vi "Setup Data.vi"(11 "?":T2={"Input Data 1D"=[], "Channel Settings"={"Supply Voltage [Vdc]"=0.0, "Max Supply Current [Idc]"=0.0, "Settling Delay"=0.0, "Temp Criteria"=0.0, "Voltage Steps [Vrms]"=[0.0, 0.25, 0.5, 1.0, 1.95, 3.0, 3.9, 5.5], "User Notes"="", "Config Wave File Path"=path "C:/ASD Power Point Beta 32J/Waveforms/150HzSine5Second.wav", "Config Voltage [Vrms]"=0.0, "Channel Configuration List"={"Channel Configuration Cluster"={"Input"=enum."---", "Enable"=FALSE, "User Notes"="", "Voltage Range"=0.0, "Current Range"=2.5}, "Channel Configuration Cluster 2"={"Input"=enum."---", "Enable"=FALSE, "User Notes"="", "Voltage Range"=0.0, "Current Range"=2.5}, "Channel Configuration Cluster 3"={"Input"=enum."---", "Enable"=FALSE, "User Notes"="", "Voltage Range"=0.0, "Current Range"=2.5}, "Channel Configuration Cluster 4"={"Input"=enum."---", "Enable"=FALSE, "User Notes"="", "Voltage Range"=0.0, "Current Range"=2.5}, "Channel Configuration Cluster 5"={"Input"=enum."---", "Enable"=FALSE, "User Notes"="", "Voltage Range"=0.0, "Current Range"=2.5}, "Channel Configuration Cluster 6"={"Input"=enum."---", "Enable"=FALSE, "User Notes"="", "Voltage Range"=0.0, "Current Range"=2.5}, "Channel Configuration Cluster 7"={"Input"=enum."---", "Enable"=FALSE, "User Notes"="", "Voltage Range"=0.0, "Current Range"=2.5}, "Channel Configuration Cluster 8"={"Input"=enum."---", "Enable"=FALSE, "User Notes"="", "Voltage Range"=0.0, "Current Range"=2.5}, "Channel Configuration Cluster 9"={"Input"=enum."---", "Enable"=FALSE, "User Notes"="", "Voltage Range"=0.0, "Current Range"=2.5}, "Channel Configuration Cluster 10"={"Input"=enum."---", "Enable"=FALSE, "User Notes"="", "Voltage Range"=0.0, "Current Range"=2.5}, "Channel Configuration Cluster 11"={"Input"=enum."---", "Enable"=FALSE, "User Notes"="", "Voltage Range"=0.0, "Current Range"=2.5}, "Channel Configuration Cluster 12"={"Input"=enum."---", "Enable"=FALSE, "User Notes"="", "Voltage Range"=0.0, "Current Range"=2.5}, "Channel Configuration Cluster 13"={"Input"=enum."---", "Enable"=FALSE, "User Notes"="", "Voltage Range"=0.0, "Current Range"=2.5}, "Channel Configuration Cluster 14"={"Input"=enum."---", "Enable"=FALSE, "User Notes"="", "Voltage Range"=0.0, "Current Range"=2.5}, "Channel Configuration Cluster 15"={"Input"=enum."---", "Enable"=FALSE, "User Notes"="", "Voltage Range"=0.0, "Current Range"=2.5}, "Channel Configuration Cluster 16"={"Input"=enum."---", "Enable"=FALSE, "User Notes"="", "Voltage Range"=0.0, "Current Range"=2.5}, "Channel Configuration Cluster 17"={"Input"=enum."---", "Enable"=FALSE, "User Notes"="", "Voltage Range"=0.0, "Current Range"=2.5}}, "User Gains"={"Gain 1"=0.0, "Gain 2"=0.0, "Gain 3"=0.0, "Gain 4"=0.0, "Gain 5"=0.0, "Gain 6"=0.0}, "Gains"={"Gain 1"=0.0, "Gain 2"=0.0, "Gain 3"=0.0, "Gain 4"=0.0, "Gain 5"=0.0, "Gain 6"=0.0}, "Gain Array"={"Gain 1"=0.0, "Gain 2"=0.0, "Gain 3"=0.0, "Gain 4"=0.0, "Gain 5"=0.0, "Gain 6"=0.0, "Gain 7"=0.0, "Gain 8"=0.0, "Gain 9"=0.0, "Gain 10"=0.0, "Gain 11"=0.0, "Gain 12"=0.0, "Gain 13"=0.0, "Gain 14"=0.0, "Gain 15"=0.0, "Gain 16"=0.0, "Gain 17"=0.0}, "Wave File Path 1"=path "", "Wave File Path 2"=path "", "Wave File Path 3"=path "", "Wave File Path 4"=path "", "Range"=FALSE, "CF"=FALSE}, "Select Data"={"Vrms Data"=FALSE, "Vpkpk Data"=FALSE, "Irms Data"=FALSE, "Power Data"=FALSE, "Ipkpk Data"=FALSE, "Temp Data"=FALSE}, "Detailed Report ?"=FALSE, "Path Settings:"={"Template Path "=path "E:/L&T Projects/Bose ASD/Excel Template/ASD Template.xltx", "Report Path"=path "E:/L&T Projects/Bose ASD/excel Reports", "JPEG1 Path "=path "C:/Users/Public/Pictures/Sample Pictures/Hydrangeas.jpg", "JPEG2 Path"=path "C:/Users/Public/Pictures/Sample Pictures/Lighthouse.jpg"}, "Vrms_Sheet"=[], "Irms_Sheet"=[], "Power_Sheet"=[], "Vpk_Sheet"=[], "Ipk_Sheet"=[], "Vrms_Avg"=[], "Irms_Avg"=[], "Power_Avg"=[], "Vpk_Avg"=[], "Ipk_Avg"=[], "Report_Ref"=refnum, "User Name"="", "Temp_Sheet"=[]} {"Channel Settings"."Gain Array"."Gain 17" format="%.2f"; "Channel Settings"."Gain Array"."Gain 16" format="%.2f"; "Channel Settings"."Gain Array"."Gain 15" format="%.2f"; "Channel Settings"."Gain Array"."Gain 14" format="%.2f"; "Channel Settings"."Gain Array"."Gain 13" format="%.2f"; "Channel Settings"."Gain Array"."Gain 12" format="%.2f"; "Channel Settings"."Gain Array"."Gain 11" format="%.2f"; "Channel Settings"."Gain Array"."Gain 10" format="%.2f"; "Channel Settings"."Gain Array"."Gain 9" format="%.2f"; "Channel Settings"."Gain Array"."Gain 8" format="%.2f"; "Channel Settings"."Gain Array"."Gain 7" format="%.2f"; "Channel Settings"."Gain Array"."Gain 6" format="%.2f"; "Channel Settings"."Gain Array"."Gain 5" format="%.2f"; "Channel Settings"."Gain Array"."Gain 4" format="%.2f"; "Channel Settings"."Gain Array"."Gain 3" format="%.2f"; "Channel Settings"."Gain Array"."Gain 2" format="%.2f"; "Channel Settings"."Gain Array"."Gain 1" format="%.2f"; "Channel Settings"."Gains"."Gain 6" format="%.2f"; "Channel Settings"."Gains"."Gain 5" format="%.2f"; "Channel Settings"."Gains"."Gain 4" format="%.2f"; "Channel Settings"."Gains"."Gain 3" format="%.2f"; "Channel Settings"."Gains"."Gain 2" format="%.2f"; "Channel Settings"."Gains"."Gain 1" format="%.2f"; "Channel Settings"."User Gains"."Gain 6" format="%.2f"; "Channel Settings"."User Gains"."Gain 5" format="%.2f"; "Channel Settings"."User Gains"."Gain 4" format="%.2f"; "Channel Settings"."User Gains"."Gain 3" format="%.2f"; "Channel Settings"."User Gains"."Gain 2" format="%.2f"; "Channel Settings"."User Gains"."Gain 1" format="%.2f"; "Channel Settings"."Channel Configuration List"."Channel Configuration Cluster 17"."Current Range" items=["1 <500m>"=0.5, "2 <1>"=1.0, "5 <2.5>"=2.5, "10 <5>"=5.0, "20 <10>"=10.0, "50 <25>"=25.0]; "Channel Settings"."Channel Configuration List"."Channel Configuration Cluster 17"."Voltage Range" items=["1.5 <0.75>"=0.75, "3 <1.5>"=1.5, "6 <3>"=3.0, "10 <5>"=5.0, "15 <7.5>"=7.5, "30 <15>"=15.0, "60 <30>"=30.0, "100 <50>"=50.0, "150 <75>"=75.0, "300 <150>"=150.0, "600 <300>"=300.0, "1000 <500>"=500.0]; "Channel Settings"."Channel Configuration List"."Channel Configuration Cluster 16"."Current Range" items=["1 <500m>"=0.5, "2 <1>"=1.0, "5 <2.5>"=2.5, "10 <5>"=5.0, "20 <10>"=10.0, "50 <25>"=25.0]; "Channel Settings"."Channel Configuration List"."Channel Configuration Cluster 16"."Voltage Range" items=["1.5 <0.75>"=0.75, "3 <1.5>"=1.5, "6 <3>"=3.0, "10 <5>"=5.0, "15 <7.5>"=7.5, "30 <15>"=15.0, "60 <30>"=30.0, "100 <50>"=50.0, "150 <75>"=75.0, "300 <150>"=150.0, "600 <300>"=300.0, "1000 <500>"=500.0]; "Channel Settings"."Channel Configuration List"."Channel Configuration Cluster 15"."Current Range" items=["1 <500m>"=0.5, "2 <1>"=1.0, "5 <2.5>"=2.5, "10 <5>"=5.0, "20 <10>"=10.0, "50 <25>"=25.0]; "Channel Settings"."Channel Configuration List"."Channel Configuration Cluster 15"."Voltage Range" items=["1.5 <0.75>"=0.75, "3 <1.5>"=1.5, "6 <3>"=3.0, "10 <5>"=5.0, "15 <7.5>"=7.5, "30 <15>"=15.0, "60 <30>"=30.0, "100 <50>"=50.0, "150 <75>"=75.0, "300 <150>"=150.0, "600 <300>"=300.0, "1000 <500>"=500.0]; "Channel Settings"."Channel Configuration List"."Channel Configuration Cluster 14"."Current Range" items=["1 <500m>"=0.5, "2 <1>"=1.0, "5 <2.5>"=2.5, "10 <5>"=5.0, "20 <10>"=10.0, "50 <25>"=25.0]; "Channel Settings"."Channel Configuration List"."Channel Configuration Cluster 14"."Voltage Range" items=["1.5 <0.75>"=0.75, "3 <1.5>"=1.5, "6 <3>"=3.0, "10 <5>"=5.0, "15 <7.5>"=7.5, "30 <15>"=15.0, "60 <30>"=30.0, "100 <50>"=50.0, "150 <75>"=75.0, "300 <150>"=150.0, "600 <300>"=300.0, "1000 <500>"=500.0]; "Channel Settings"."Channel Configuration List"."Channel Configuration Cluster 13"."Current Range" items=["1 <500m>"=0.5, "2 <1>"=1.0, "5 <2.5>"=2.5, "10 <5>"=5.0, "20 <10>"=10.0, "50 <25>"=25.0]; "Channel Settings"."Channel Configuration List"."Channel Configuration Cluster 13"."Voltage Range" items=["1.5 <0.75>"=0.75, "3 <1.5>"=1.5, "6 <3>"=3.0, "10 <5>"=5.0, "15 <7.5>"=7.5, "30 <15>"=15.0, "60 <30>"=30.0, "100 <50>"=50.0, "150 <75>"=75.0, "300 <150>"=150.0, "600 <300>"=300.0, "1000 <500>"=500.0]; "Channel Settings"."Channel Configuration List"."Channel Configuration Cluster 12"."Current Range" items=["1 <500m>"=0.5, "2 <1>"=1.0, "5 <2.5>"=2.5, "10 <5>"=5.0, "20 <10>"=10.0, "50 <25>"=25.0]; "Channel Settings"."Channel Configuration List"."Channel Configuration Cluster 12"."Voltage Range" items=["1.5 <0.75>"=0.75, "3 <1.5>"=1.5, "6 <3>"=3.0, "10 <5>"=5.0, "15 <7.5>"=7.5, "30 <15>"=15.0, "60 <30>"=30.0, "100 <50>"=50.0, "150 <75>"=75.0, "300 <150>"=150.0, "600 <300>"=300.0, "1000 <500>"=500.0]; "Channel Settings"."Channel Configuration List"."Channel Configuration Cluster 11"."Current Range" items=["1 <500m>"=0.5, "2 <1>"=1.0, "5 <2.5>"=2.5, "10 <5>"=5.0, "20 <10>"=10.0, "50 <25>"=25.0]; "Channel Settings"."Channel Configuration List"."Channel Configuration Cluster 11"."Voltage Range" items=["1.5 <0.75>"=0.75, "3 <1.5>"=1.5, "6 <3>"=3.0, "10 <5>"=5.0, "15 <7.5>"=7.5, "30 <15>"=15.0, "60 <30>"=30.0, "100 <50>"=50.0, "150 <75>"=75.0, "300 <150>"=150.0, "600 <300>"=300.0, "1000 <500>"=500.0]; "Channel Settings"."Channel Configuration List"."Channel Configuration Cluster 10"."Current Range" items=["1 <500m>"=0.5, "2 <1>"=1.0, "5 <2.5>"=2.5, "10 <5>"=5.0, "20 <10>"=10.0, "50 <25>"=25.0]; "Channel Settings"."Channel Configuration List"."Channel Configuration Cluster 10"."Voltage Range" items=["1.5 <0.75>"=0.75, "3 <1.5>"=1.5, "6 <3>"=3.0, "10 <5>"=5.0, "15 <7.5>"=7.5, "30 <15>"=15.0, "60 <30>"=30.0, "100 <50>"=50.0, "150 <75>"=75.0, "300 <150>"=150.0, "600 <300>"=300.0, "1000 <500>"=500.0]; "Channel Settings"."Channel Configuration List"."Channel Configuration Cluster 9"."Voltage Range" items=["1.5 <0.75>"=0.75, "3 <1.5>"=1.5, "6 <3>"=3.0, "10 <5>"=5.0, "15 <7.5>"=7.5, "30 <15>"=15.0, "60 <30>"=30.0, "100 <50>"=50.0, "150 <75>"=75.0, "300 <150>"=150.0, "600 <300>"=300.0, "1000 <500>"=500.0]; "Channel Settings"."Channel Configuration List"."Channel Configuration Cluster 9"."Current Range" items=["10m <5m>"=0.005, "20m <10m>"=0.01, "50m <25m>"=0.025, "100m <50m>"=0.05, "200m <100m>"=0.1, "500m <250m>"=0.25, "1 <500m>"=0.5, "2 <1>"=1.0, "5 <2.5>"=2.5]; "Channel Settings"."Channel Configuration List"."Channel Configuration Cluster 8"."Voltage Range" items=["1.5 <0.75>"=0.75, "3 <1.5>"=1.5, "6 <3>"=3.0, "10 <5>"=5.0, "15 <7.5>"=7.5, "30 <15>"=15.0, "60 <30>"=30.0, "100 <50>"=50.0, "150 <75>"=75.0, "300 <150>"=150.0, "600 <300>"=300.0, "1000 <500>"=500.0]; "Channel Settings"."Channel Configuration List"."Channel Configuration Cluster 8"."Current Range" items=["10m <5m>"=0.005, "20m <10m>"=0.01, "50m <25m>"=0.025, "100m <50m>"=0.05, "200m <100m>"=0.1, "500m <250m>"=0.25, "1 <500m>"=0.5, "2 <1>"=1.0, "5 <2.5>"=2.5]; "Channel Settings"."Channel Configuration List"."Channel Configuration Cluster 7"."Voltage Range" items=["1.5 <0.75>"=0.75, "3 <1.5>"=1.5, "6 <3>"=3.0, "10 <5>"=5.0, "15 <7.5>"=7.5, "30 <15>"=15.0, "60 <30>"=30.0, "100 <50>"=50.0, "150 <75>"=75.0, "300 <150>"=150.0, "600 <300>"=300.0, "1000 <500>"=500.0]; "Channel Settings"."Channel Configuration List"."Channel Configuration Cluster 7"."Current Range" items=["10m <5m>"=0.005, "20m <10m>"=0.01, "50m <25m>"=0.025, "100m <50m>"=0.05, "200m <100m>"=0.1, "500m <250m>"=0.25, "1 <500m>"=0.5, "2 <1>"=1.0, "5 <2.5>"=2.5]; "Channel Settings"."Channel Configuration List"."Channel Configuration Cluster 6"."Voltage Range" items=["1.5 <0.75>"=0.75, "3 <1.5>"=1.5, "6 <3>"=3.0, "10 <5>"=5.0, "15 <7.5>"=7.5, "30 <15>"=15.0, "60 <30>"=30.0, "100 <50>"=50.0, "150 <75>"=75.0, "300 <150>"=150.0, "600 <300>"=300.0, "1000 <500>"=500.0]; "Channel Settings"."Channel Configuration List"."Channel Configuration Cluster 6"."Current Range" items=["10m <5m>"=0.005, "20m <10m>"=0.01, "50m <25m>"=0.025, "100m <50m>"=0.05, "200m <100m>"=0.1, "500m <250m>"=0.25, "1 <500m>"=0.5, "2 <1>"=1.0, "5 <2.5>"=2.5]; "Channel Settings"."Channel Configuration List"."Channel Configuration Cluster 5"."Voltage Range" items=["1.5 <0.75>"=0.75, "3 <1.5>"=1.5, "6 <3>"=3.0, "10 <5>"=5.0, "15 <7.5>"=7.5, "30 <15>"=15.0, "60 <30>"=30.0, "100 <50>"=50.0, "150 <75>"=75.0, "300 <150>"=150.0, "600 <300>"=300.0, "1000 <500>"=500.0]; "Channel Settings"."Channel Configuration List"."Channel Configuration Cluster 5"."Current Range" items=["10m <5m>"=0.005, "20m <10m>"=0.01, "50m <25m>"=0.025, "100m <50m>"=0.05, "200m <100m>"=0.1, "500m <250m>"=0.25, "1 <500m>"=0.5, "2 <1>"=1.0, "5 <2.5>"=2.5]; "Channel Settings"."Channel Configuration List"."Channel Configuration Cluster 4"."Voltage Range" items=["1.5 <0.75>"=0.75, "3 <1.5>"=1.5, "6 <3>"=3.0, "10 <5>"=5.0, "15 <7.5>"=7.5, "30 <15>"=15.0, "60 <30>"=30.0, "100 <50>"=50.0, "150 <75>"=75.0, "300 <150>"=150.0, "600 <300>"=300.0, "1000 <500>"=500.0]; "Channel Settings"."Channel Configuration List"."Channel Configuration Cluster 4"."Current Range" items=["10m <5m>"=0.005, "20m <10m>"=0.01, "50m <25m>"=0.025, "100m <50m>"=0.05, "200m <100m>"=0.1, "500m <250m>"=0.25, "1 <500m>"=0.5, "2 <1>"=1.0, "5 <2.5>"=2.5]; "Channel Settings"."Channel Configuration List"."Channel Configuration Cluster 3"."Voltage Range" items=["1.5 <0.75>"=0.75, "3 <1.5>"=1.5, "6 <3>"=3.0, "10 <5>"=5.0, "15 <7.5>"=7.5, "30 <15>"=15.0, "60 <30>"=30.0, "100 <50>"=50.0, "150 <75>"=75.0, "300 <150>"=150.0, "600 <300>"=300.0, "1000 <500>"=500.0]; "Channel Settings"."Channel Configuration List"."Channel Configuration Cluster 3"."Current Range" items=["10m <5m>"=0.005, "20m <10m>"=0.01, "50m <25m>"=0.025, "100m <50m>"=0.05, "200m <100m>"=0.1, "500m <250m>"=0.25, "1 <500m>"=0.5, "2 <1>"=1.0, "5 <2.5>"=2.5]; "Channel Settings"."Channel Configuration List"."Channel Configuration Cluster 2"."Voltage Range" items=["1.5 <0.75>"=0.75, "3 <1.5>"=1.5, "6 <3>"=3.0, "10 <5>"=5.0, "15 <7.5>"=7.5, "30 <15>"=15.0, "60 <30>"=30.0, "100 <50>"=50.0, "150 <75>"=75.0, "300 <150>"=150.0, "600 <300>"=300.0, "1000 <500>"=500.0]; "Channel Settings"."Channel Configuration List"."Channel Configuration Cluster 2"."Current Range" items=["10m <5m>"=0.005, "20m <10m>"=0.01, "50m <25m>"=0.025, "100m <50m>"=0.05, "200m <100m>"=0.1, "500m <250m>"=0.25, "1 <500m>"=0.5, "2 <1>"=1.0, "5 <2.5>"=2.5]; "Channel Settings"."Channel Configuration List"."Channel Configuration Cluster"."Voltage Range" items=["1.5 <0.75>"=0.75, "3 <1.5>"=1.5, "6 <3>"=3.0, "10 <5>"=5.0, "15 <7.5>"=7.5, "30 <15>"=15.0, "60 <30>"=30.0, "100 <50>"=50.0, "150 <75>"=75.0, "300 <150>"=150.0, "600 <300>"=300.0, "1000 <500>"=500.0]; "Channel Settings"."Channel Configuration List"."Channel Configuration Cluster"."Current Range" items=["10m <5m>"=0.005, "20m <10m>"=0.01, "50m <25m>"=0.025, "100m <50m>"=0.05, "200m <100m>"=0.1, "500m <250m>"=0.25, "1 <500m>"=0.5, "2 <1>"=1.0, "5 <2.5>"=2.5]; "Channel Settings"."Settling Delay" min=0.0 format="%<%H:%M:%S>t"; "Input Data 1D"."WT1800 Averages"."Vrms" format="%.3f"; "Input Data 1D"."WT1800 Averages"."Irms" format="%.3f"; "Input Data 1D"."WT1800 Averages"."Power" format="%.3f"; "Input Data 1D"."WT1800 Averages"."Vpkpk" format="%.3f"; "Input Data 1D"."WT1800 Averages"."Ipkpk" format="%.3f"; "Input Data 1D"."WT1800 Measurements"."Vrms" format="%.3f"; "Input Data 1D"."WT1800 Measurements"."Irms" format="%.3f"; "Input Data 1D"."WT1800 Measurements"."Power" format="%.3f"; "Input Data 1D"."WT1800 Measurements"."Vpkpk" format="%.3f"; "Input Data 1D"."WT1800 Measurements"."Ipkpk" format="%.3f"; "Input Data 1D"."DSA Averages"."Vrms" format="%.3f"; "Input Data 1D"."DSA Averages"."Vdc" format="%.3f"; "Input Data 1D"."DSA Averages"."Vpk+" format="%.3f"; "Input Data 1D"."DSA Averages"."Vpk-" format="%.3f"; "Input Data 1D"."DSA Averages"."Vpkpk" format="%.3f"; "Input Data 1D"."DSA Measurements"."Vrms" format="%.3f"; "Input Data 1D"."DSA Measurements"."Vdc" format="%.3f"; "Input Data 1D"."DSA Measurements"."Vpk+" format="%.3f"; "Input Data 1D"."DSA Measurements"."Vpk-" format="%.3f"; "Input Data 1D"."DSA Measurements"."Vpkpk" format="%.3f"}) -> (3 "Set up data":string[][][](array[string]))   [LabVIEW 2021]
uses:
  Datalog Controls/Data.ctl
  <vilib>/Utility/NIReport.llb/NI_report.lvclass
  Controls/Datalog Cluster Array.ctl
  Controls/Datalog Bundle Control.ctl
  Controls/WT1800 Functions.ctl
  Controls/WT1800 Measurements.ctl
  Controls/WT1800 Readings.ctl
  Controls/DSA Functions.ctl
  Controls/DSA Measurements.ctl
  Controls/DSA Readings.ctl
  Controls/Settings Control.ctl
  Controls/Channel Configuration List.ctl
  Controls/Channel Configuration Cluster.ctl
  Controls/Channel Configuration Cluster High Current.ctl
  Controls/Gain Averages.ctl
  Controls/Gain Array.ctl
  Datalog Controls/Select_Data.ctl
panel:
  out "Input":T1(ring)
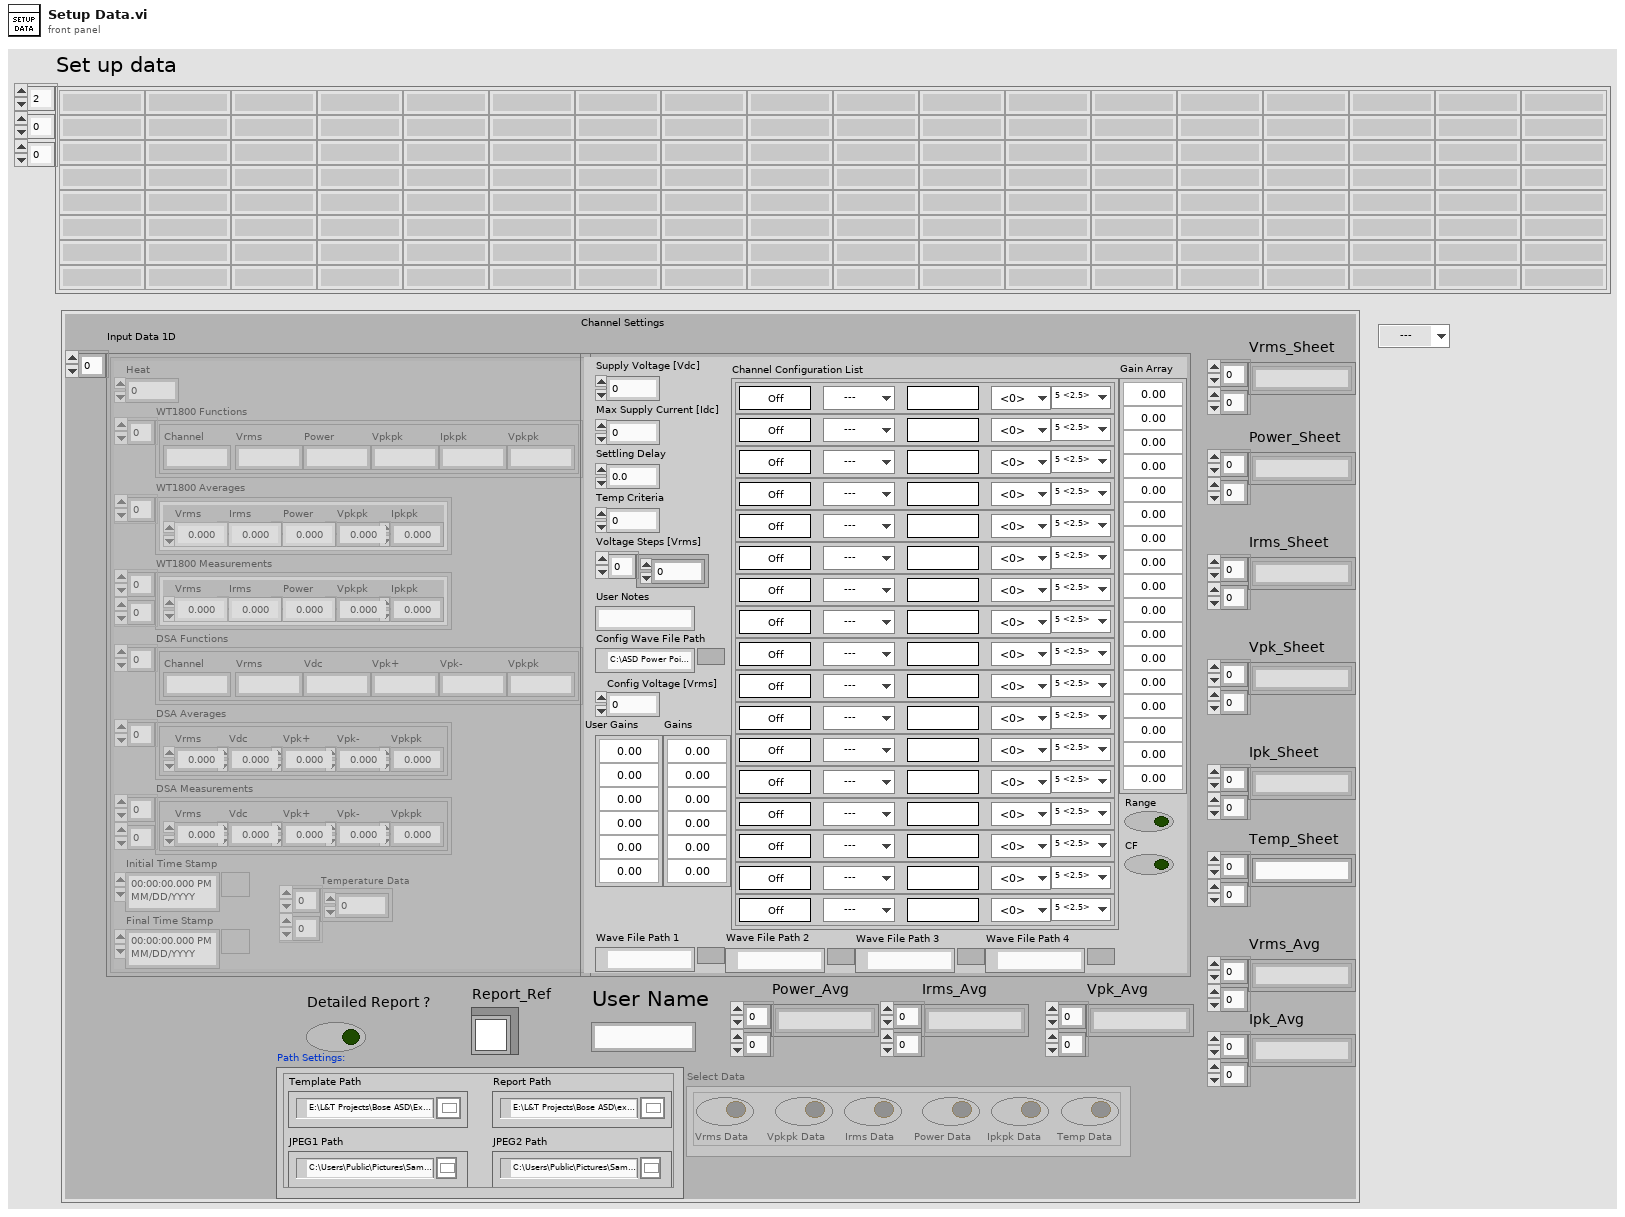
[diagram p1: front panel]
types:
  T1 = enum16{"---", "1", "1 AVG", "2", "2 AVG", "3", "3 AVG", "4", "4 AVG"}
  T2 = typedef "Data.ctl" = cluster{"Input Data 1D":T3, "Channel Settings":T11, "Select Data":T17, "Detailed Report ?":bool, "Path Settings:":cluster{"Template Path ":path, "Report Path":path, "JPEG1 Path ":path, "JPEG2 Path":path}, "Vrms_Sheet":string[][], "Irms_Sheet":string[][], "Power_Sheet":string[][], "Vpk_Sheet":string[][], "Ipk_Sheet":string[][], "Vrms_Avg":string[][], "Irms_Avg":string[][], "Power_Avg":string[][], "Vpk_Avg":string[][], "Ipk_Avg":string[][], "Report_Ref":refnum<class "NI_report.lvclass">, "User Name":string, "Temp_Sheet":string[][]}
  T3 = typedef "Datalog Cluster Array.ctl" = T4[]
  T4 = typedef "Datalog Bundle Control.ctl" = cluster{"Heat":dbl, "WT1800 Functions":T5, "WT1800 Averages":T6, "WT1800 Measurements":T7[][], "DSA Functions":T8, "DSA Averages":T9, "DSA Measurements":T10[][], "Initial Time Stamp":timestamp, "Final Time Stamp":timestamp, "Temperature Data":sgl[][]}
  T5 = typedef "WT1800 Functions.ctl" = cluster{"Channel":string, "Vrms":string, "Power":string, "Vpkpk":string, "Ipkpk":string, "Vpkpk":string}[]
  T6 = typedef "WT1800 Measurements.ctl" = T7[]
  T7 = typedef "WT1800 Readings.ctl" = cluster{"Vrms":sgl, "Irms":sgl, "Power":sgl, "Vpkpk":sgl, "Ipkpk":sgl}
  T8 = typedef "DSA Functions.ctl" = cluster{"Channel":string, "Vrms":string, "Vdc":string, "Vpk+":string, "Vpk-":string, "Vpkpk":string}[]
  T9 = typedef "DSA Measurements.ctl" = T10[]
  T10 = typedef "DSA Readings.ctl" = cluster{"Vrms":sgl, "Vdc":sgl, "Vpk+":sgl, "Vpk-":sgl, "Vpkpk":sgl}
  T11 = typedef "Settings Control.ctl" = cluster{"Supply Voltage [Vdc]":sgl, "Max Supply Current [Idc]":sgl, "Settling Delay":dbl, "Temp Criteria":sgl, "Voltage Steps [Vrms]":sgl[], "User Notes":string, "Config Wave File Path":path, "Config Voltage [Vrms]":sgl, "Channel Configuration List":T12, "User Gains":T15, "Gains":T15, "Gain Array":T16, "Wave File Path 1":path, "Wave File Path 2":path, "Wave File Path 3":path, "Wave File Path 4":path, "Range":bool, "CF":bool}
  T12 = typedef "Channel Configuration List.ctl" = cluster{"Channel Configuration Cluster":T13, "Channel Configuration Cluster 2":T13, "Channel Configuration Cluster 3":T13, "Channel Configuration Cluster 4":T13, "Channel Configuration Cluster 5":T13, "Channel Configuration Cluster 6":T13, "Channel Configuration Cluster 7":T13, "Channel Configuration Cluster 8":T13, "Channel Configuration Cluster 9":T13, "Channel Configuration Cluster 10":T14, "Channel Configuration Cluster 11":T14, "Channel Configuration Cluster 12":T14, "Channel Configuration Cluster 13":T14, "Channel Configuration Cluster 14":T14, "Channel Configuration Cluster 15":T14, "Channel Configuration Cluster 16":T14, "Channel Configuration Cluster 17":T14}
  T13 = typedef "Channel Configuration Cluster.ctl" = cluster{"Input":enum16{"---", "1", "1 AVG", "2", "2 AVG", "3", "3 AVG", "4", "4 AVG"}, "Enable":bool, "User Notes":string, "Voltage Range":dbl, "Current Range":dbl}
  T14 = typedef "Channel Configuration Cluster High Current.ctl" = cluster{"Input":enum16{"---", "1", "1 AVG", "2", "2 AVG", "3", "3 AVG", "4", "4 AVG"}, "Enable":bool, "User Notes":string, "Voltage Range":dbl, "Current Range":dbl}
  T15 = typedef "Gain Averages.ctl" = cluster{"Gain 1":dbl, "Gain 2":dbl, "Gain 3":dbl, "Gain 4":dbl, "Gain 5":dbl, "Gain 6":dbl}
  T16 = typedef "Gain Array.ctl" = cluster{"Gain 1":dbl, "Gain 2":dbl, "Gain 3":dbl, "Gain 4":dbl, "Gain 5":dbl, "Gain 6":dbl, "Gain 7":dbl, "Gain 8":dbl, "Gain 9":dbl, "Gain 10":dbl, "Gain 11":dbl, "Gain 12":dbl, "Gain 13":dbl, "Gain 14":dbl, "Gain 15":dbl, "Gain 16":dbl, "Gain 17":dbl}
  T17 = typedef "Select_Data.ctl" = cluster{"Vrms Data":bool, "Vpkpk Data":bool, "Irms Data":bool, "Power Data":bool, "Ipkpk Data":bool, "Temp Data":bool}
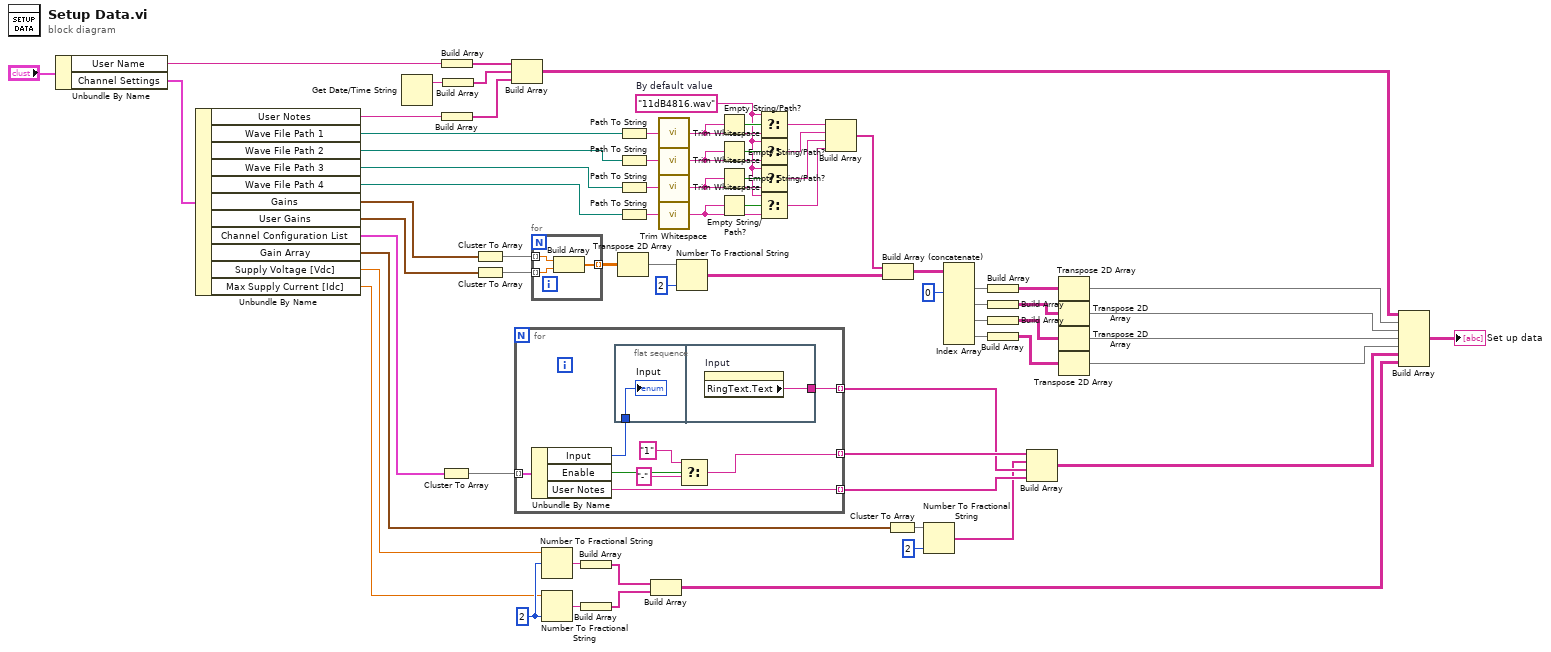
[diagram p0: block diagram]
diagram:
  w9 = "11dB4816.wav"  # By default value
  w43 = i16 2 ("width (-)")
  n1 = Unbundle By Name("?") -> ("User Name"=w60:string, "Channel Settings"=w59:T11)
  n2 = Unbundle By Name(w59) -> ("User Notes"=w44:string, "Wave File Path 1"=w64:path, "Wave File Path 2"=w12:path, "Wave File Path 3"=w11:path, "Wave File Path 4"=w10:path, "Gains"=w30:T15, "User Gains"=w26:T15, "Channel Configuration List"=w35:T12, "Gain Array"=w34:T16, "Supply Voltage [Vdc]"=w42:sgl, "Max Supply Current [Idc]"=w41:sgl)
  n3 = Get Date/Time String() -> (date string=w66:string)  [unwired: 3 in, 1 out]
  n4 = Cluster To Array(cluster=w35) -> (array=w62:T14[])
  n5 = Build Array(w60) -> (w65:string[])
  n6 = Build Array(w44) -> (w68:string[])
  n7 = Build Array(w66) -> (w67:string[])
  n8 = Cluster To Array(cluster=w30) -> (array=w28:dbl[])
  n9 = Cluster To Array(cluster=w26) -> (array=w29:dbl[])
  n10 = Build Array(w65, w67, w68) -> (w47:string[][])
  n11 = for {
    tunnel: w62 -> [w80] mode=indexing
    tunnel: [w73] -> w40 mode=indexing
    tunnel: [w79] -> w63 mode=indexing
    tunnel: [w74] -> w54 mode=indexing
    n12 = Unbundle By Name(w80) -> ("Input"=w78:T1, "Enable"=w77:bool, "User Notes"=w79:string)
    n13 = flat-sequence {
      tunnel: w78 -> [w81]
      tunnel: [w82] -> w73
      frame #0 {
        "Input" <- w81
      }
      frame #1 {
        n14 = property on="Input" class="Enum (strict)"() -> ("RingText.Text"=w82:string)  [unwired: 2 in, 2 out]
      }
    }
    n15 = Select(t="1", s=w77, f="-") -> (s? t:f=w74:string)
  }
  n16 = for {
    tunnel: w29 -> [w85] mode=indexing
    tunnel: w28 -> [w84] mode=indexing
    tunnel: [w83] -> w27 mode=indexing
    n17 = Build Array(w84, w85) -> (w83:dbl[])
  }
  n18 = Number To Fractional String(number=w42, width (-)=w43) -> (F-format string=w71:string)  [unwired: 2 in]
  n19 = Number To Fractional String(number=w41, precision (6)=w43) -> (F-format string=w69:string)  [unwired: 2 in]
  n20 = Build Array(w71) -> (w72:string[])
  n21 = Build Array(w69) -> (w70:string[])
  n22 = Transpose 2D Array(2D array=w27) -> (transposed array=w55:dbl[][])
  n23 = Path To String(path=w64) -> (string=w57:string)
  n24 = Path To String(path=w12) -> (string=w20:string)
  n25 = Path To String(path=w11) -> (string=w17:string)
  n26 = Path To String(path=w10) -> (string=w14:string)
  n27 = Build Array(w72, w70) -> (w46:string[][])
  n28 = call <vilib>:"Trim Whitespace.vi"("string"=w57) -> ("trimmed string"=w56:string)  [unwired: 1 in]
  n29 = call <vilib>:"Trim Whitespace.vi"("string"=w20) -> ("trimmed string"=w19:string)  [unwired: 1 in]
  n30 = call <vilib>:"Trim Whitespace.vi"("string"=w17) -> ("trimmed string"=w16:string)  [unwired: 1 in]
  n31 = call <vilib>:"Trim Whitespace.vi"("string"=w14) -> ("trimmed string"=w13:string)  [unwired: 1 in]
  n32 = Number To Fractional String(number=w55, precision (6)=i16 2) -> (F-format string=w6:string[][])  [unwired: 2 in]
  n33 = Empty String/Path?(string/path=w56) -> (empty?=w58:bool)
  n34 = Empty String/Path?(string/path=w19) -> (empty?=w21:bool)
  n35 = Empty String/Path?(string/path=w16) -> (empty?=w18:bool)
  n36 = Empty String/Path?(string/path=w13) -> (empty?=w15:bool)
  n37 = Select(t=w9, s=w58, f=w56) -> (s? t:f=w8:string)
  n38 = Select(t=w9, s=w21, f=w19) -> (s? t:f=w5:string)
  n39 = Select(t=w9, s=w18, f=w16) -> (s? t:f=w4:string)
  n40 = Select(t=w9, s=w15, f=w13) -> (s? t:f=w3:string)
  n41 = Build Array(w8, w5, w4, w3) -> (w7:string[])
  n42 = Build Array (concatenate)(w7, w6) -> (w48:string[][])
  n43 = Cluster To Array(cluster=w34) -> (array=w37:dbl[])
  n44 = Number To Fractional String(number=w37, precision (6)=i16 2) -> (F-format string=w36:string[])  [unwired: 2 in]
  n45 = Index Array(array=w48, index (col) #1=0 ("disabled index (col)")) -> (element #1=w52:string[], element #2=w50:string[], element #3=w24:string[], element #4=w22:string[])  [unwired: 7 in]
  n46 = Build Array(w52) -> (w51:string[][])
  n47 = Build Array(w50) -> (w49:string[][])
  n48 = Build Array(w24) -> (w25:string[][])
  n49 = Build Array(w22) -> (w23:string[][])
  n50 = Build Array(w54, w36, w40, w63) -> (w31:string[][])
  n51 = Transpose 2D Array(2D array=w51) -> (transposed array=w33:string[][])
  n52 = Transpose 2D Array(2D array=w49) -> (transposed array=w32:string[][])
  n53 = Transpose 2D Array(2D array=w25) -> (transposed array=w2:string[][])
  n54 = Transpose 2D Array(2D array=w23) -> (transposed array=w1:string[][])
  n55 = Build Array(w47, w33, w32, w2, w1, w31, w46) -> (→"Set up data":string[][][])
